vi "getDAQmx_Config.vi"(8 "error in (no error)":errorcluster, 11 "DAQmx in":refnum<class "DAQmx.lvclass">) -> (0 "error out":errorcluster, 2 "DAQmx.Config":T1={"Buffer Size (S)"=10, "Master Slave"=enum."MASTER"}, 3 "DAQmx out":refnum<class "DAQmx.lvclass">)   [LabVIEW 2020, in "DAQmx.lvclass"]
uses:
  DAQmx.lvclass
  Type Defs/DAQmx_Config.ctl
  DAQmx.lvclass/DAQmx.ctl
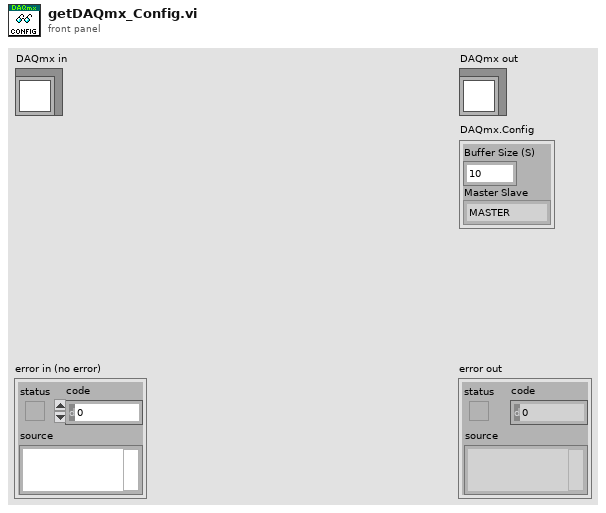
[diagram p1: front panel]
types:
  T1 = typedef "DAQmx.lvclass/DAQmx_Config.ctl" = cluster{"Buffer Size (S)":i32, "Master Slave":enum16{"MASTER", "SLAVE"}}
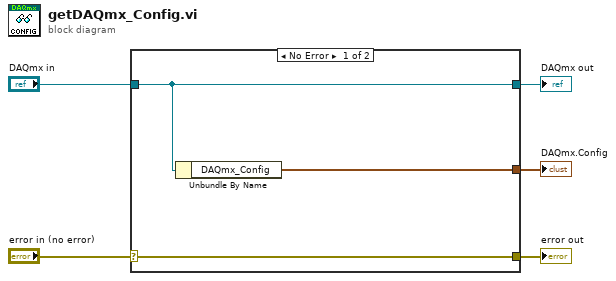
[diagram p0: block diagram]
diagram:
  n1 = case shown="No Error" "error in (no error)" {
    selector: "error in (no error)" -> [w8 w9]
    tunnel: [w8 w9] -> w4
    tunnel: [w7 w10] -> w2
    tunnel: "DAQmx in" -> [w7 w10]
    tunnel: [w6 _] -> w1
    frame No Error {
      n2 = Unbundle By Name(w7) -> ("DAQmx_Config"=w6:T1)
    }
    frame Error {
    }
  }
  "error out" <- w4
  "DAQmx out" <- w2
  "DAQmx.Config" <- w1
